vi "onStart.vi"(8 "error in (no error)":errorcluster, 11 "Server in":refnum<class "Server.lvclass">) -> (0 "error out":errorcluster, 3 "Server out":refnum<class "Server.lvclass">)   [LabVIEW 2013, in "MQTT Server.lvlib" / "Server.lvclass"]
uses:
  Server.lvclass
  MQTT_Base/Base Class/MQTT_Base.lvclass
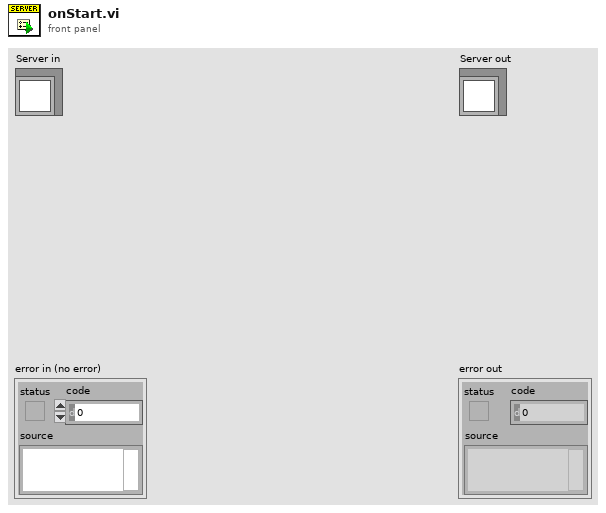
[diagram p1: front panel]
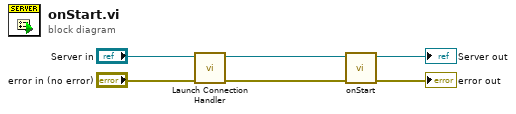
[diagram p0: block diagram]
diagram:
  n1 = call "Launch Connection Handler.vi"("error in (no error)"="error in (no error)", "Server in"="Server in") -> ("error out"=w2:errorcluster, "Server out"=w3:refnum<class "Server.lvclass">)  [unwired: 8 in]
  n2 = call-parent "onStart.vi"("error in (no error)"=w2, "MQTT_Base in"=w3) -> ("error out"=→"error out":errorcluster, "MQTT_Base out"=→"Server out":refnum<class "Server.lvclass">)  [unwired: 8 in]
